vi "Ballast.vi"(11 "Full System Configuration":T1 {"Ballast"."Side" max=5 step=1; "Ballast"."Small" max=5 step=1; "Ballast"."Main" max=5 step=1}) -> (3 "Array":T5[](array[typedef]))   [LabVIEW 2023]
uses:
  Option Type Defs/Rack.ctl
  Option Type Defs/Parts List.ctl
  Option Type Defs/Middle Rail.ctl
  Option Type Defs/Ballast.ctl
  Option Type Defs/Full System Configuration.ctl
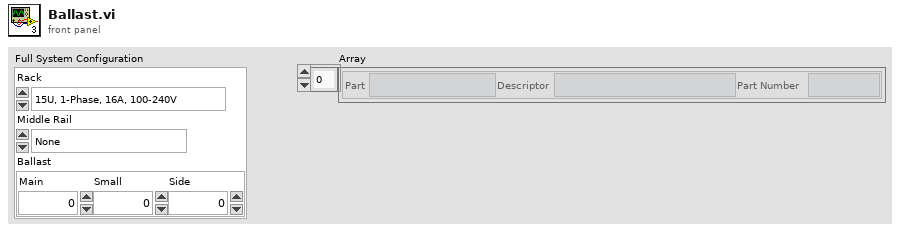
[diagram p1: front panel]
types:
  T1 = typedef "Full System Configuration.ctl" = cluster{"Rack":T2, "Middle Rail":T3, "Ballast":T4}
  T2 = typedef "Rack.ctl" = enum16{"15U, 1-Phase, 16A, 100-240V", "15U, 1-Phase, 24A, 100-240V", "38U, 3-Phase Delta, 50A, 200-240V", "38U, 1-Phase, 24A, 100-120V", "38U, 3-Phase Wye, 50A, 200-240V", "38U, 3-Phase Delta, 50A, 380-480V", "38U, 3-Phase Delta, 32A, 200-240V", "38U, 3-Phase Wye, 16A, 100-240V", "44U, 1-Phase, 24A, 100-240V", "44U, 3-Phase Delta, 32A, 200-240V"}
  T3 = typedef "Middle Rail.ctl" = enum16{"None", "Flip Side Rear, D=168.83mm", "Parallel Rear, D=145mm", "Flip Side Front, D=145mm", "Parallel Front, D=145mm"}
  T4 = typedef "Ballast.ctl" = cluster{"Main":u16, "Small":u16, "Side":u16}
  T5 = typedef "Parts List.ctl" = cluster{"Part":string, "Descriptor":string, "Part Number":string}
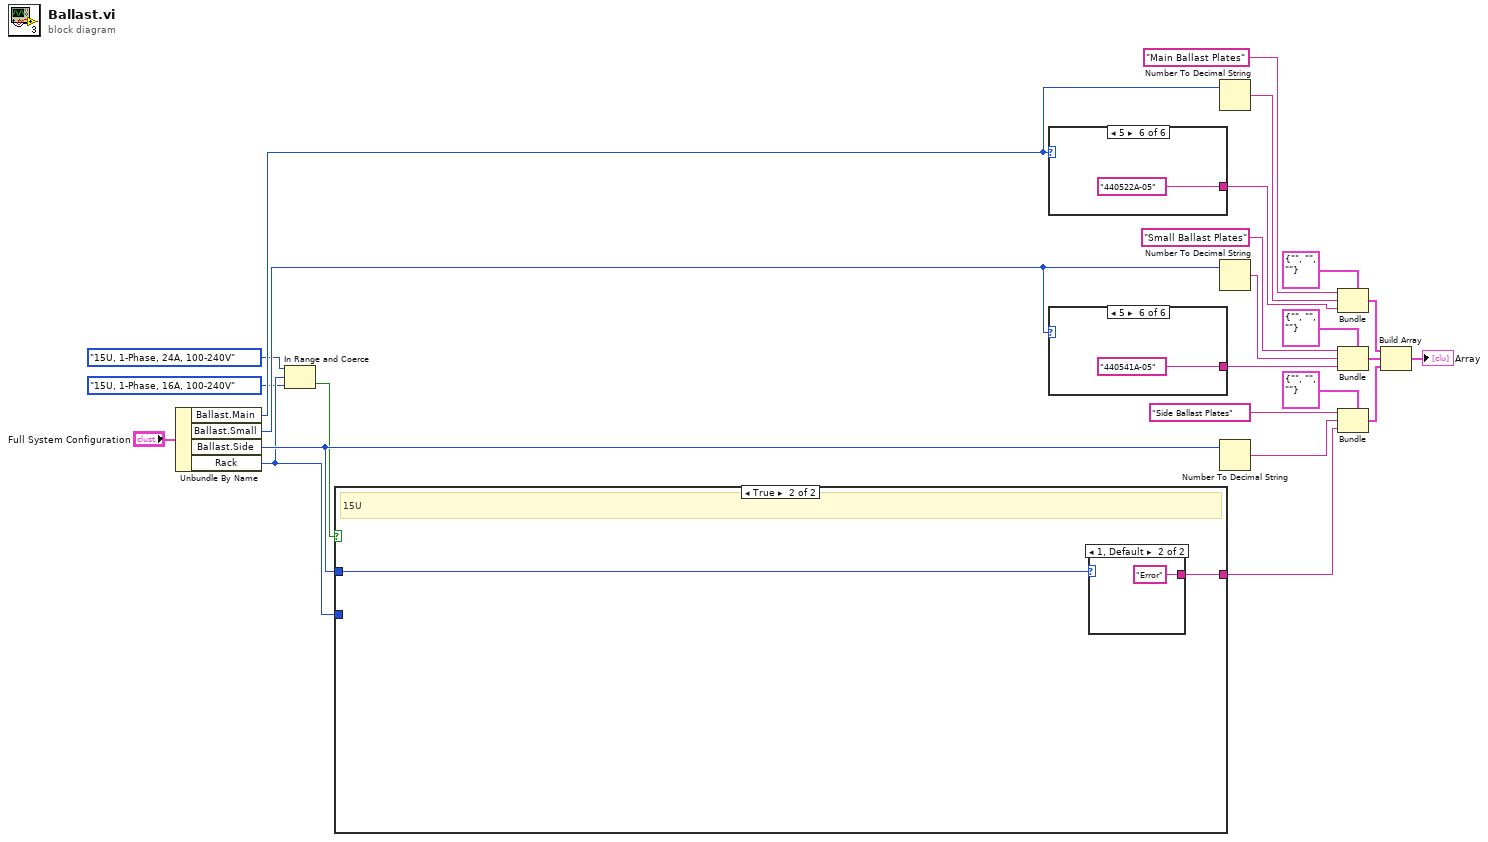
[diagram p0: block diagram]
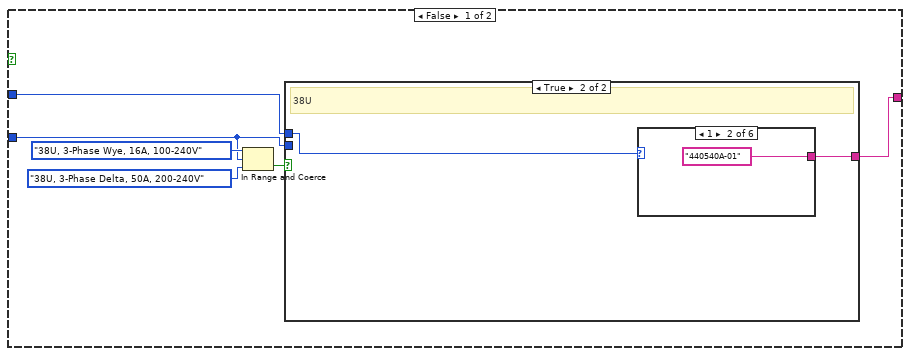
[diagram p2: hidden frame]
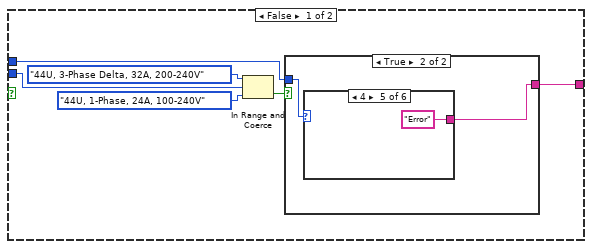
[diagram p3: hidden frame]
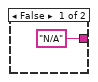
[diagram p4: hidden frame]
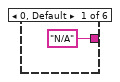
[diagram p5: hidden frame]
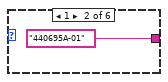
[diagram p6: hidden frame]
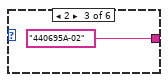
[diagram p7: hidden frame]
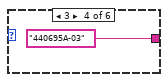
[diagram p8: hidden frame]
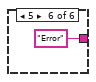
[diagram p9: hidden frame]
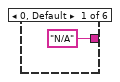
[diagram p10: hidden frame]
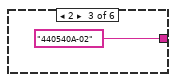
[diagram p11: hidden frame]
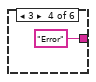
[diagram p12: hidden frame]
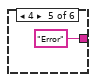
[diagram p13: hidden frame]
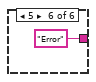
[diagram p14: hidden frame]
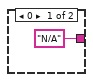
[diagram p15: hidden frame]
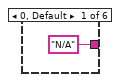
[diagram p16: hidden frame]
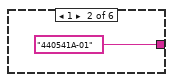
[diagram p17: hidden frame]
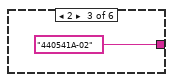
[diagram p18: hidden frame]
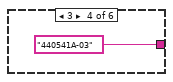
[diagram p19: hidden frame]
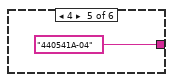
[diagram p20: hidden frame]
diagram:
  n1 = Unbundle By Name("Full System Configuration") -> ("Ballast.Main"=w16:u16, "Ballast.Small"=w19:u16, "Ballast.Side"=w24:u16, "Rack"=w5:T2)
  n2 = In Range and Coerce(upper limit=Rack."15U, 1-Phase, 24A, 100-240V" ("Rack"), x=w5, lower limit=Rack."15U, 1-Phase, 16A, 100-240V" ("Rack")) -> (In Range?=w4:bool)  [unwired: 1 out]
  n3 = case shown="True" w4 {
    tunnel: [w30 w55] -> w12
    tunnel: w5 -> [w26 _]
    tunnel: w24 -> [w25 w54]
    frame False {
      n4 = In Range and Coerce(upper limit=Rack."38U, 3-Phase Wye, 16A, 100-240V" ("Rack"), x=w26, lower limit=Rack."38U, 3-Phase Delta, 50A, 200-240V" ("Rack")) -> (In Range?=w27:bool)  [unwired: 1 out]
      n5 = case shown="True" w27 {
        tunnel: [w32 w47] -> w30
        tunnel: w26 -> [w34 _]
        tunnel: w25 -> [w31 w46]
        frame False {
          n6 = In Range and Coerce(upper limit=Rack."44U, 3-Phase Delta, 32A, 200-240V" ("Rack"), x=w34, lower limit=Rack."44U, 1-Phase, 24A, 100-240V" ("Rack")) -> (In Range?=w33:bool)  [unwired: 1 out]
          n7 = case shown="True" w33 {
            tunnel: ["N/A" w39] -> w32
            tunnel: w31 -> [_ w38]
            frame False {
            }
            frame True {
              n8 = case shown="4" w38 {
                tunnel: ["N/A" "440695A-01" "440695A-02" "440695A-03" "Error" "Error"] -> w39
                frame 0, Default {
                }
                frame 1 {
                }
                frame 2 {
                }
                frame 3 {
                }
                frame 4 {
                }
                frame 5 {
                }
              }
            }
          }
        }
        frame True {
          # "38U"
          n9 = case shown="1" w46 {
            tunnel: ["N/A" "440540A-01" "440540A-02" "Error" "Error" "Error"] -> w47
            frame 0, Default {
            }
            frame 1 {
            }
            frame 2 {
            }
            frame 3 {
            }
            frame 4 {
            }
            frame 5 {
            }
          }
        }
      }
    }
    frame True {
      # "15U"
      n10 = case shown="1, Default" w54 {
        tunnel: ["N/A" "Error"] -> w55
        frame 0 {
        }
        frame 1, Default {
        }
      }
    }
  }
  n11 = case shown="5" w16 {
    tunnel: ["N/A" "440522A-01" "440522A-02" "440522A-03" "440522A-04" "440522A-05"] -> w9
    frame 0, Default {
    }
    frame 1 {
    }
    frame 2 {
    }
    frame 3 {
    }
    frame 4 {
    }
    frame 5 {
    }
  }
  n12 = case shown="5" w19 {
    tunnel: ["N/A" "440541A-01" "440541A-02" "440541A-03" "440541A-04" "440541A-05"] -> w11
    frame 0, Default {
    }
    frame 1 {
    }
    frame 2 {
    }
    frame 3 {
    }
    frame 4 {
    }
    frame 5 {
    }
  }
  n13 = Number To Decimal String(number=w16) -> (decimal integer string=w17:string)  [unwired: 1 in]
  n14 = Number To Decimal String(number=w19) -> (decimal integer string=w21:string)  [unwired: 1 in]
  n15 = Number To Decimal String(number=w24) -> (decimal integer string=w23:string)  [unwired: 1 in]
  n16 = Bundle(cluster=T5 {"Part"="", "Descriptor"="", "Part Number"=""}, "Part"="Main Ballast Plates", "Descriptor"=w17, "Part Number"=w9) -> (w10:T5)
  n17 = Bundle(cluster=T5 {"Part"="", "Descriptor"="", "Part Number"=""}, "Part"="Small Ballast Plates", "Descriptor"=w21, "Part Number"=w11) -> (w13:T5)
  n18 = Bundle(cluster=T5 {"Part"="", "Descriptor"="", "Part Number"=""}, "Part"="Side Ballast Plates", "Descriptor"=w23, "Part Number"=w12) -> (w14:T5)
  n19 = Build Array(w10, w13, w14) -> (→"Array":T5[])
